vi "Pre Launch Init.vi"(11 "Measurement Generator in":refnum<class "Measurement Generator.lvclass">) -> (0 "error out":errorcluster, 3 "Measurement Generator out":refnum<class "Measurement Generator.lvclass">)   [LabVIEW 2020, in "Measurement Generator.lvclass"]
doc: "(<B>Filename</B>: Actor Framework.lvlib:Actor.lvclass:Pre Launch Init.vi)\n\nDefines behavior that occurs after the Launch Nested Actor method is invoked but before the actor's Actor Core method begins running.\n\nBy default, this method does nothing. A descendant class may override it to define behavior."
uses:
  Measurement Generator.lvclass
  <vilib>/ActorFramework/Actor/Actor.lvclass
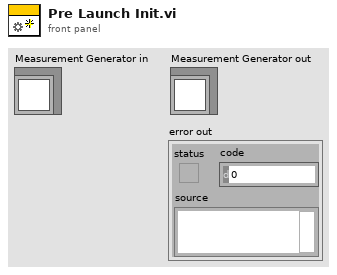
[diagram p1: front panel]
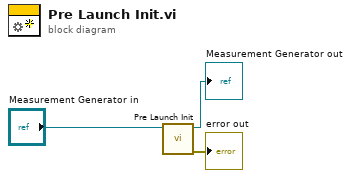
[diagram p0: block diagram]
diagram:
  n1 = call-parent "Pre Launch Init.vi"("Actor in"="Measurement Generator in") -> ("error out"=→"error out":errorcluster, "Actor out"=→"Measurement Generator out":refnum<class "Measurement Generator.lvclass">)  [unwired: 9 in]
